vi "jitterHold.vi"(7 "jitterChanged?":bool, 8 "Y-jitter":dbl, 9 "X-jitter":dbl, 11 "Array":cluster{"Array":dbl[], "Array":dbl[]}[](array[cluster])) -> (3 "Array 2":cluster{"Array":dbl[], "Array":dbl[]}[](array[cluster]))   [LabVIEW 2013]
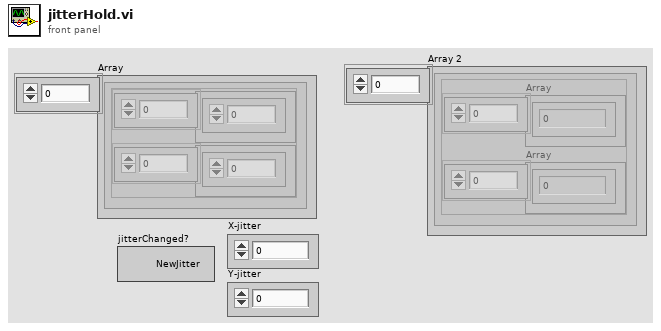
[diagram p1: front panel]
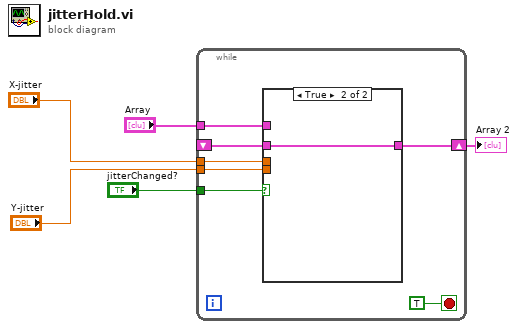
[diagram p0: block diagram]
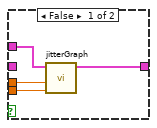
[diagram p2: hidden frame]
diagram:
  n1 = while {
    shift-right: [w11] -> w4
    shift-left: _ -> [w12]
    tunnel: "jitterChanged?" -> [w9]
    tunnel: "X-jitter" -> [w8]
    tunnel: "Y-jitter" -> [w7]
    tunnel: "Array" -> [w6]
    stop <- TRUE stop-if-true
    n2 = case shown="True" w9 {
      tunnel: w12 -> [_ w17]
      tunnel: [w16 w17] -> w11
      tunnel: w8 -> [w15 _]
      tunnel: w7 -> [w14 _]
      tunnel: w6 -> [w13 _]
      frame False {
        n3 = call "jitterGraph.vi"("Y-jitter"=w14, "X-jitter"=w15, "GraphPlots"=w13) -> ("jitteredGraphPlots"=w16:cluster{"Array":dbl[], "Array":dbl[]}[])  [unwired: 8 in]
      }
      frame True {
      }
    }
  }
  "Array 2" <- w4
